vi "Launch Module.vi"(8 "error in (no error)":errorcluster, 9 "params":variant, 11 "Controller in":refnum<class "Controller.lvclass">) -> (0 "error out":errorcluster, 3 "Controller out":refnum<class "Controller.lvclass">)   [LabVIEW 2020, in "Controller.lvlib" / "Controller.lvclass"]
uses:
  Controller.lvclass
  Controller.lvclass/Controller.ctl
  RPC/TypeDefs/Request.ctl
  Properties/Read Response.vi
  Properties/Read E-Stop.vi
  Properties/Read Globals.vi
  <vilib>/ErrorRing/Error Ring.xnode
  RPC.lvlib
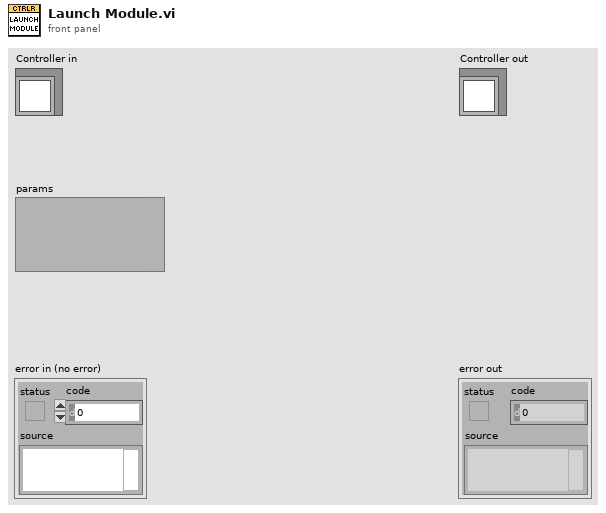
[diagram p1: front panel]
types:
  T1 = typedef "RPC.lvlib/Request.ctl" = cluster{"Method":string, "Params":variant}
  T2 = cluster{"Module Info[0]":string, "Module Info[1]":string}
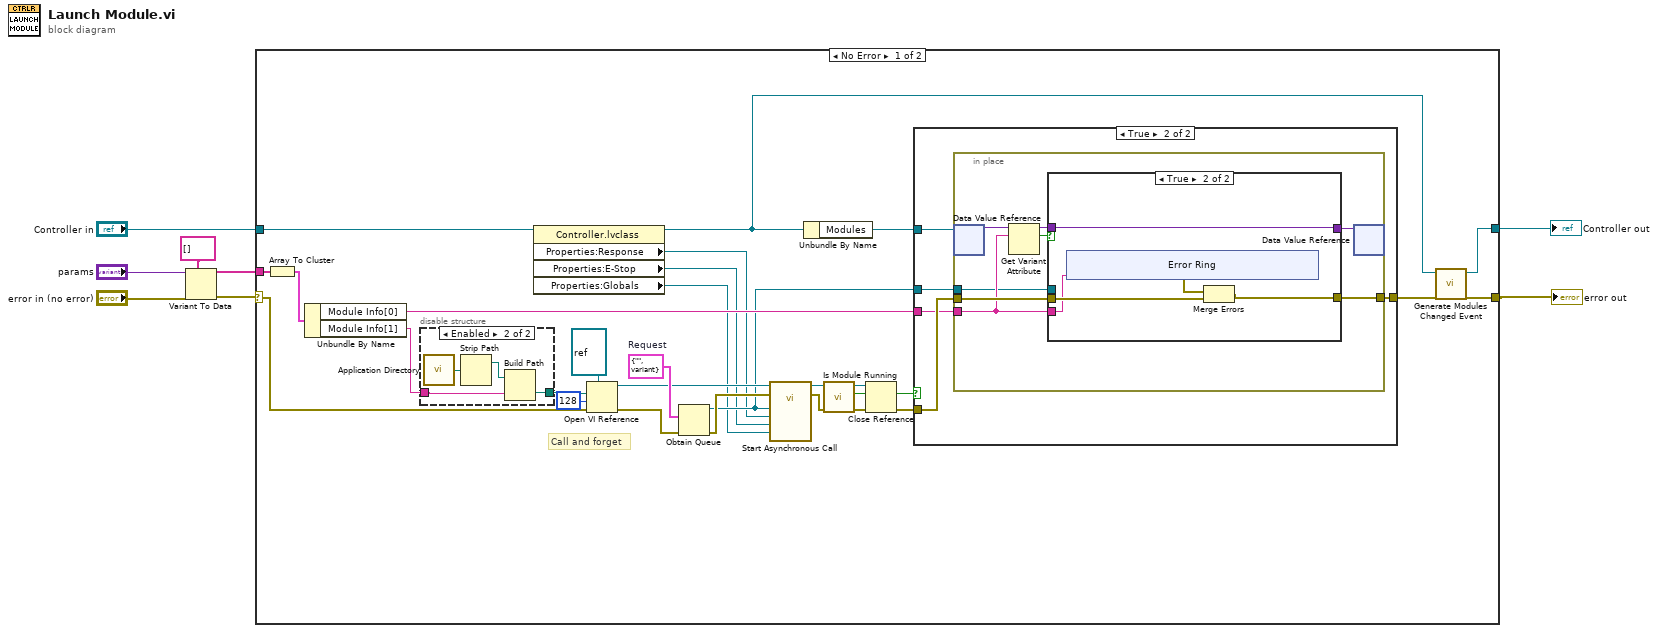
[diagram p0: block diagram]
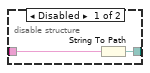
[diagram p2: hidden frame]
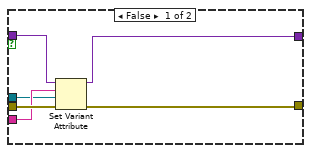
[diagram p4: hidden frame]
diagram:
  n1 = Variant To Data(error in="error in (no error)", type=string[] [] ("Module Info"), Variant="params") -> (data=w4:string[], error out=w5:errorcluster)
  n2 = case shown="No Error" w5 {
    selector: w5 -> [w25 w74]
    tunnel: "Controller in" -> [w24 w73]
    tunnel: w4 -> [w23 _]
    tunnel: [w10 w74] -> w1
    tunnel: [w11 w73] -> w2
    frame No Error {
      w32 = T1 {"Method"="", "Params"=variant}  # Request
      # "Call and forget"
      n3 = Array To Cluster(array=w23) -> (cluster=w22:T2)
      n4 = Unbundle By Name(w22) -> ("Module Info[0]"=w18:string, "Module Info[1]"=w21:string)
      n5 = disable-structure shown="Enabled" {
        disable-tunnel: [w38 w41] -> w36
        disable-tunnel: w21 -> [w37 w42]
        frame Disabled {
          n6 = String To Path(string=w37) -> (path=w38:path)
        }
        frame Enabled {
          n7 = call <vilib>:"Application Directory.vi"() -> ("Application Directory"=w40:path)
          n8 = Strip Path(path=w40) -> (stripped path=w39:path)  [unwired: 1 out]
          n9 = Build Path(base path=w39, name or relative path=w42) -> (appended path=w41:path)
        }
      }
      n10 = property class="Controller.lvclass"(reference=w24) -> (reference out=w9:refnum<class "Controller.lvclass">, "Properties:Response"=w16:refnum<user-event>, "Properties:E-Stop"=w15:refnum<user-event>, "Properties:Globals"=w14:refnum<data-value>)  [unwired: 1 in, 1 out]
      n11 = Open VI Reference(type specifier VI Refnum (for type only)=refnum<vi> refnum, vi path=w36, options=128, error in (no error)=w25) -> (vi reference=w31:refnum<vi>, error out=w33:errorcluster)  [unwired: 2 in]
      n12 = Obtain Queue(element data type=w32, error in (no error)=w33) -> (queue out=w17:refnum<queue>, error out=w19:errorcluster)  [unwired: 3 in, 1 out]
      n13 = call-by-ref "Start Asynchronous Call"(reference=w31, error in=w19, "Globals"=w14, "E-Stop"=w15, "Response"=w16, "RequestMQ"=w17) -> (reference out=w20:refnum<vi>, error out=w26:errorcluster)  [unwired: 8 in]
      n14 = Unbundle By Name(w9) -> ("Modules"=w13:refnum<data-value>)
      n15 = call "Is Module Running.vi"("error in (no error)"=w26, "VI reference in"=w20) -> ("error out"=w29:errorcluster, "Is Running?"=w27:bool, "VI reference out"=w28:refnum<vi>)  [unwired: 6 in, 1 out]
      n16 = Close Reference(reference=w28, error in (no error)=w29) -> (error out=w35:errorcluster)
      n17 = case shown="True" w27 {
        tunnel: w35 -> [w43 w48]
        tunnel: [w43 w47] -> w12
        tunnel: w18 -> [_ w46]
        tunnel: w17 -> [_ w45]
        tunnel: w13 -> [_ w44]
        frame False {
        }
        frame True {
          n18 = in-place {
            in-place-border: w46 -> [w52]
            in-place-border: w48 -> [w55]
            in-place-border: w45 -> [w51]
            in-place-border: [w54] -> w47
            n19 = in-place-dvr #1(w44) -> (w53:variant)  [unwired: 1 out]
            n20 = Get Variant Attribute(Variant=w53, name=w52) -> (duplicate Variant=w50:variant, found=w49:bool)  [unwired: 2 in, 2 out]
            n21 = case shown="True" w49 {
              tunnel: [w62 w67] -> w56
              tunnel: w55 -> [w61 w65]
              tunnel: [w57 w66] -> w54
              tunnel: w52 -> [w60 w64]
              tunnel: w51 -> [w59 _]
              tunnel: w50 -> [w58 w67]
              frame False {
                n22 = Set Variant Attribute(Variant=w58, name=w60, value=w59, error in=w61) -> (Variant out=w62:variant, error out=w57:errorcluster)  [unwired: 1 out]
              }
              frame True {
                n23 = xnode "Error Ring"("parameter 0"=w64) -> ("error out"=w63:errorcluster)
                n24 = Merge Errors(w63, w65) -> (w66:errorcluster)
              }
            }
            n25 = in-place-dvr #1(w56) -> ()  [unwired: 2 out]
          }
        }
      }
      n26 = call "Generate Modules Changed Event.vi"("error in (no error)"=w12, "Controller in"=w9) -> ("error out"=w10:errorcluster, "Controller out"=w11:refnum<class "Controller.lvclass">)  [unwired: 8 in]
    }
    frame Error {
    }
  }
  "error out" <- w1
  "Controller out" <- w2
